vi "Acceleration Sensor-Direct.vi"() -> ()   [LabVIEW 2009]
uses:
  <vilib>/NXT/Block Support/NXT_InputPort.ctl
  <vilib>/NXT/Subs/LVHSConnector.ctl
panel:
  in  "stop":bool
  out "Z":i16(knob) scale=-2000.0..2000.0
  out "Y":i16(knob) scale=-2000.0..2000.0
  out "X":i16(knob) scale=-2000.0..2000.0
  out "X":i16(slide)=-128 scale=-35.0..35.0
  out "Z":i16(slide)=-128 caption="Y" scale=-35.0..35.0
  out "Y":i16(slide)=-128 scale=-35.0..35.0
  out "Z":i16(slide)=-128 caption="X" scale=-35.0..35.0
  out "Y":i16(slide)=-128 scale=-35.0..35.0
  out "X":i16(slide)=-128 scale=-35.0..35.0
  out "Z":dbl
  out "Y":dbl
  out "X":dbl
  out "Z":dbl=-128.0
  out "Y":dbl=-128.0
  out "X":dbl=-128.0
  out "NXT dup":T1={"error"={"status"=FALSE, "code"=0, "source"=""}, "address"="", "NXT #"=-1, "Show Error"=TRUE} caption="NXT"
  in  "NXT":T1={"error"={"status"=FALSE, "code"=0, "source"=""}, "address"="", "NXT #"=-1, "Show Error"=TRUE}
  in  "Input Port":T2 items=["Port 1", "Port 2", "Port 3", "Port 4"]
  # "Tilt"
  # "Acceleration"
  # "mindsensors.com\nCopyright (c) 2009 by mindsensors.com\nEmail: info (<at>) mindsensors (<dot>) com\n\nThis program is free software. You can redistribute it and/or modify\nit under the terms of the GNU General Public License as published by\nthe Free Software Foundation; version 3 of the License.\nRead the license at: http://www.gnu.org/licenses/gpl.txt"
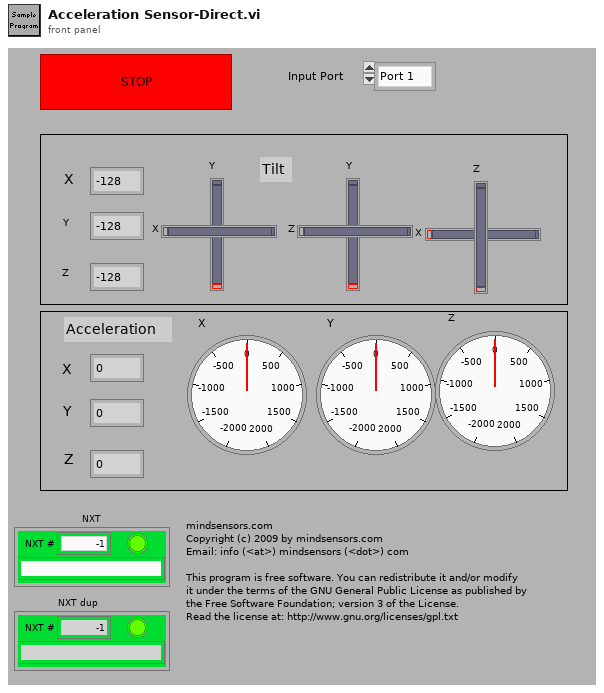
[diagram p1: front panel]
types:
  T1 = typedef "LVHSConnector.ctl" = cluster{"error":errorcluster, "address":string, "NXT #":i32, "Show Error":bool}
  T2 = typedef "NXT_InputPort.ctl" = u8
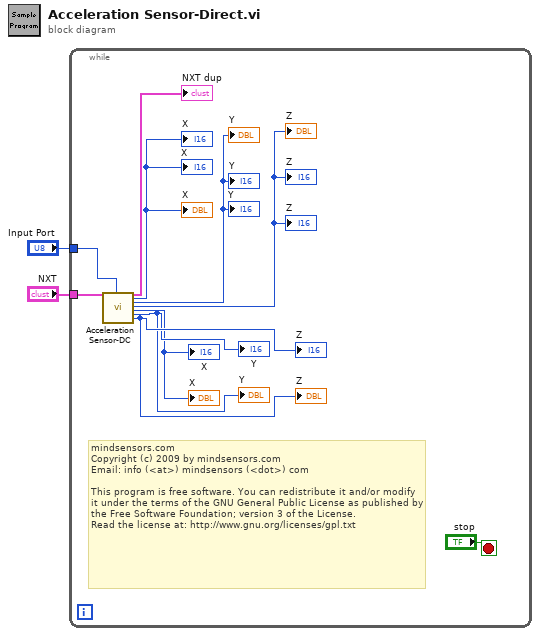
[diagram p0: block diagram]
diagram:
  n1 = while {
    tunnel: "Input Port" -> [w12]
    tunnel: "NXT" -> [w11]
    stop <- "stop" stop-if-true
    # "mindsensors.com\nCopyright (c) 2009 by mindsensors.com\nEmail: info (<at>) mindsensors (<dot>) com\n\nThis program is free software. You can redistribute it and/or modify\nit under the terms of the GNU General Public License as published by\nthe Free Software Foundation; version 3 of the License.\nRead the license at: http://www.gnu.org/licenses/gpl.txt"
    n2 = call "Acceleration Sensor-DC.vi"("NXT"=w11, "Input Port"=w12) -> ("NXT dup"=→"NXT dup":T1, "X Tilt"=→"X" →"X" →"X":i16, "Y Tilt"=→"Y" →"Y" →"Y":i16, "Z Tilt"=→"Z" →"Z" →"Z":i16, "X Accel"=→"X" →"X":i16, "Y Accel"=→"Y" →"Y":i16, "Z Accel"=→"Z" →"Z":i16)  [unwired: 18 in, 1 out]
  }
